vi "BeamWidthPage.vi"() -> ()   [LabVIEW 2026]
panel:
  in  "PRINT":bool
  in  "Beam X Measurement":T1
  in  "Cluster 5":T2
  in  "Enter Chosen Beam X Length into table below":string[][](table) caption="Transducer Information"
  in  "Beam Profile":string(combo)
  out "Beam Width Graph":cluster{"timebase":dbl[], "data":u16[]}[](graph)
  out "Axis Controls 2":T3
  in  "E-Stop Reset 2":bool
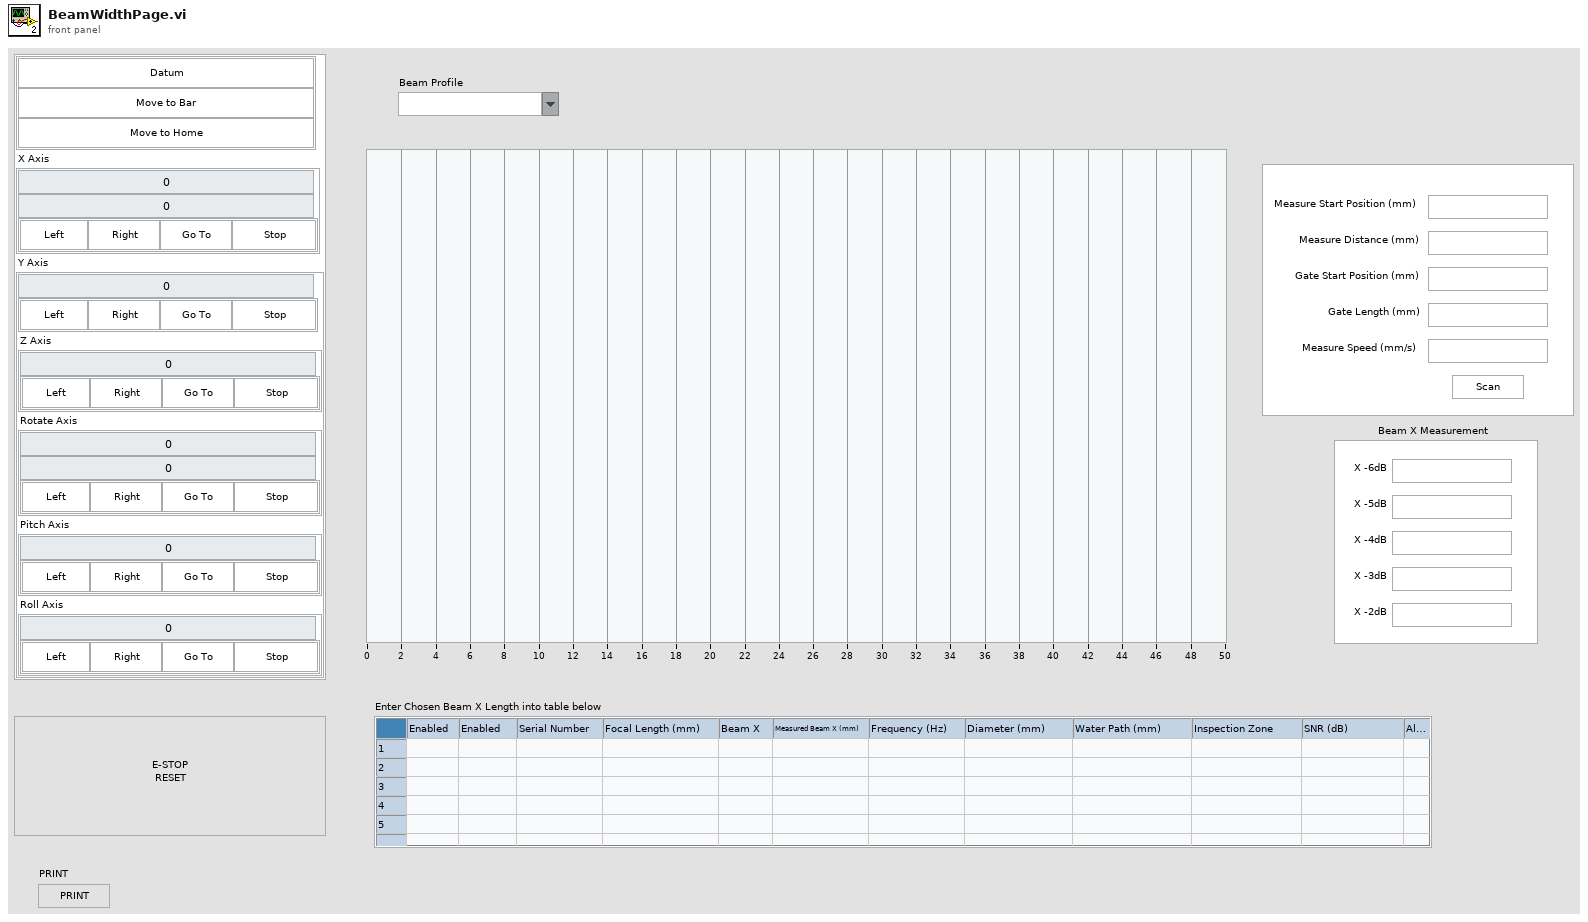
[diagram p1: front panel]
types:
  T1 = cluster{"X -6dB":string, "X -5dB":string, "X -4dB":string, "X -3dB":string, "X -2dB":string}
  T2 = cluster{"Measure Start Position (mm)":string, "Measure Distance (mm)":string, "Gate Start Position (mm)":string, "Gate Length (mm)":string, "Measure Speed (mm/s)":string, "Button 2":bool}
  T3 = cluster{"Buttons":cluster{"Datum":bool, "Move to Bar":bool, "Move to Home":bool}, "X Axis":cluster{"Calculated X Value":dbl, "Encoder X Value":dbl, "X Axis Movement Buttons":cluster{"Left":bool, "Right":bool, "Go To":bool, "Stop":bool}}, "Y Axis":cluster{"Encoder Y Value":dbl, "Y Axis Movement Buttons":cluster{"Left":bool, "Right":bool, "Go To":bool, "Stop":bool}, "Z Axis":cluster{"Encoder Z Value":dbl, "Z Axis Movement Buttons":cluster{"Left":bool, "Right":bool, "Go To":bool, "Stop":bool}}, "Rotate Axis":cluster{"Calculated Rotate Value":dbl, "Encoder Rotate Value":dbl, "Rotate Axis Movement Buttons":cluster{"Left":bool, "Right":bool, "Go To":bool, "Stop":bool}}, "Pitch Axis":cluster{"Encoder Pitch Value":dbl, "Pitch Axis Movement Buttons":cluster{"Left":bool, "Right":bool, "Go To":bool, "Stop":bool}}, "Roll Axis":cluster{"Encoder Roll Value":dbl, "Roll Axis Movement Buttons":cluster{"Left":bool, "Right":bool, "Go To":bool, "Stop":bool}}}}
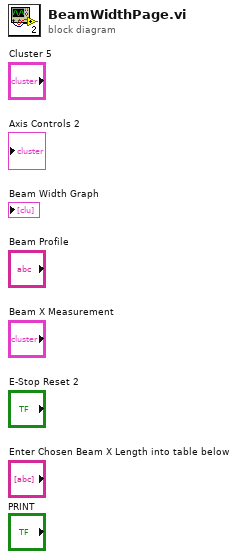
[diagram p0: block diagram]
diagram:
